vi "RPM Ramp.vi"(10 "Requested RPM":dbl, 11 "Current RPM":dbl) -> (3 "RPM Ramp":dbl[](array[numeric]))   [LabVIEW 2017]
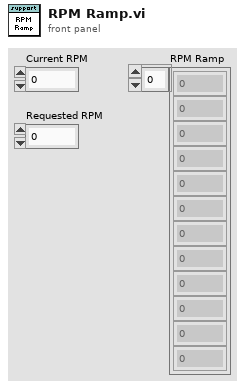
[diagram p1: front panel]
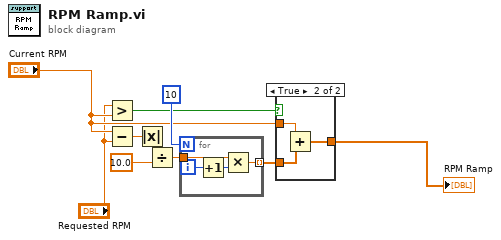
[diagram p0: block diagram]
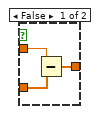
[diagram p2: hidden frame]
diagram:
  n1 = Greater?(x="Requested RPM", y="Current RPM") -> (0:w2:bool)
  n2 = Subtract(x="Current RPM", y="Requested RPM") -> (x-y=w4:dbl)
  n3 = Absolute Value(x=w4) -> (abs(x)=w5:dbl)
  n4 = Divide(x=w5, y=10.0) -> (x/y=w7:dbl)
  n5 = for {
    N: 10 -> [_]
    tunnel: w7 -> [w13]
    tunnel: [w12] -> w8 mode=indexing
    i -> [w14]
    n6 = Increment(x=w14) -> (x+1=w11:i32)
    n7 = Multiply(x=w13, y=w11) -> (x*y=w12:dbl)
  }
  n8 = case shown="True" w2 {
    tunnel: [w17 w20] -> w1
    tunnel: w8 -> [w16 w19]
    tunnel: "Current RPM" -> [w15 w18]
    frame False {
      n9 = Subtract(x=w15, y=w16) -> (x-y=w17:dbl[])
    }
    frame True {
      n10 = Add(x=w18, y=w19) -> (x+y=w20:dbl[])
    }
  }
  "RPM Ramp" <- w1
